vi "ShopAssistantAnswer.vi"(8 "error in (no error)":errorcluster, 11 "ShopAssistant in":refnum<class "ShopAssistant.lvclass">) -> (0 "error out":errorcluster, 3 "ShopAssistant out":refnum<class "ShopAssistant.lvclass">)   [LabVIEW 2020, in "ShopAssistant.lvlib" / "ShopAssistant.lvclass"]
uses:
  ShopAssistant.lvclass
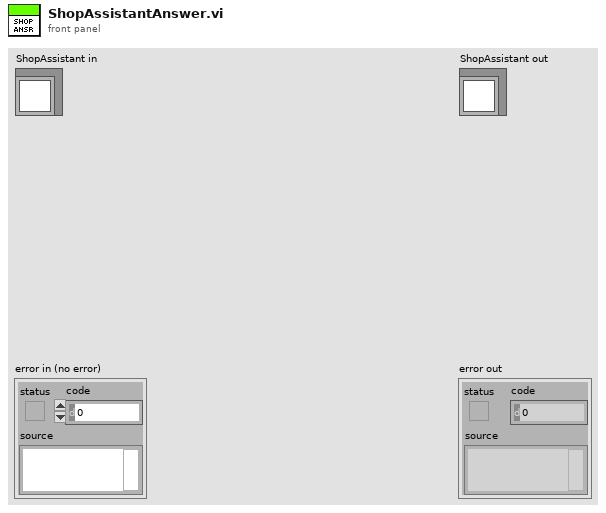
[diagram p1: front panel]
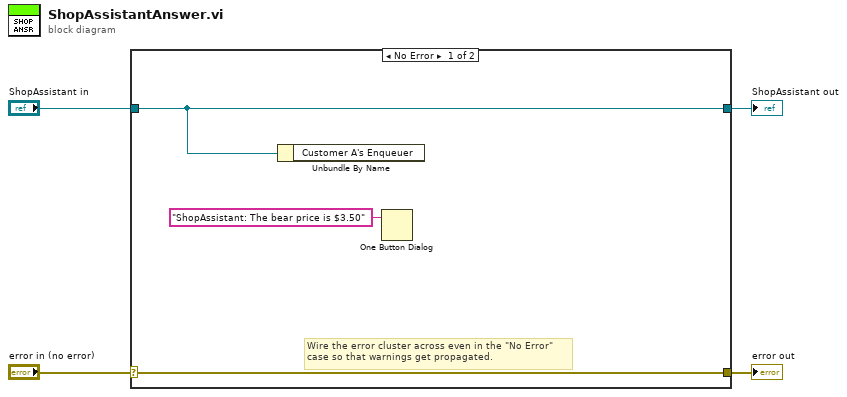
[diagram p0: block diagram]
diagram:
  n1 = case shown="No Error" "error in (no error)" {
    selector: "error in (no error)" -> [w7 w9]
    tunnel: [w7 w9] -> w3
    tunnel: [w5 w8] -> w1
    tunnel: "ShopAssistant in" -> [w5 w8]
    frame No Error {
      # "Wire the error cluster across even in the \"No Error\"\ncase so that warnings get propagated."
      n2 = Unbundle By Name(w5) -> ()  [unwired: 1 out]
      n3 = One Button Dialog(message="ShopAssistant: The bear price is $3.50") -> ()  [unwired: 1 in, 1 out]
    }
    frame Error {
    }
  }
  "error out" <- w3
  "ShopAssistant out" <- w1
